vi "I Value (Read).vi"(6 "ISOBUS address":T1=-1 caption="ISOBUS address (-1)", 8 "error in":errorcluster, 11 "Mercury Reference In":T4) -> (0 "error out":errorcluster, 1 "Unit":T2, 2 "I Value":dbl min=0.0 max=100.0 format="%#.1g", 3 "Mercury Reference Out":T4, 4 "Valid?":T3)   [LabVIEW 2013, in "Mercury iXX.lvlib" / "Control Loop.lvlib"]
doc: "Check the I value of the PID associated with control loop."
uses:
  Control Loop.lvlib
  Mercury iXX.lvlib
  Private/Controls/Command Verbs.ctl
  Controls/Unit String.ctl
  Controls/Is Valid LED.ctl
  Controls/Comms Transport Layer.ctl
  Private/Controls/Query Dynamic Reference.ctl
  Controls/Mercury Reference.ctl
  Controls/ISOBus Address.ctl
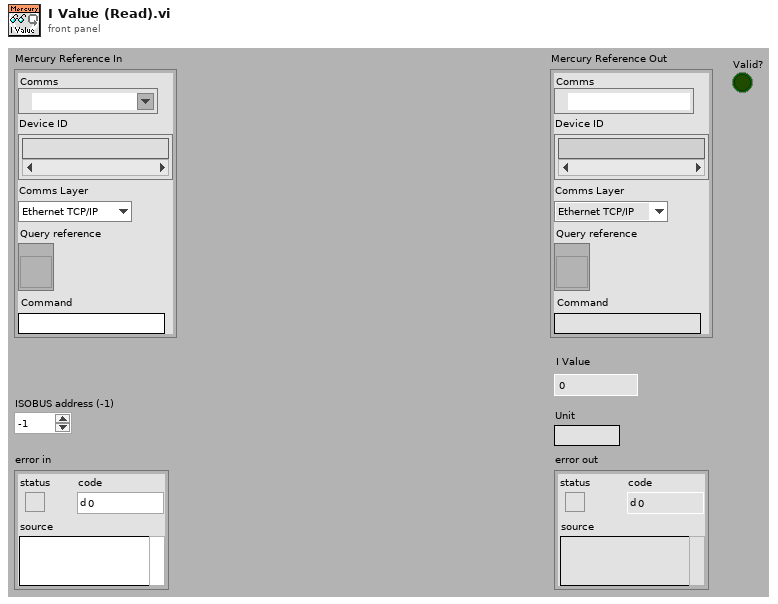
[diagram p1: front panel]
types:
  T1 = typedef "Mercury iXX.lvlib/ISOBus Address.ctl" = i32
  T2 = typedef "Mercury iXX.lvlib/Unit String.ctl" = string
  T3 = typedef "Mercury iXX.lvlib/Is Valid LED.ctl" = bool
  T4 = typedef "Mercury iXX.lvlib/Mercury Reference.ctl" = cluster{"Comms":refnum<visa-resource-name>, "Device ID":string[], "Comms Layer":T5, "Command":string, "Query reference":T6}
  T5 = typedef "Mercury iXX.lvlib/Comms Transport Layer.ctl" = enum16{"Ethernet TCP/IP", "USB", "ISOBus - RS-232", "GPIB"}
  T6 = typedef "Mercury iXX.lvlib/Query Dynamic Reference.ctl" = refnum<vi>
  T7 = typedef "Mercury iXX.lvlib/Command Verbs.ctl" = string
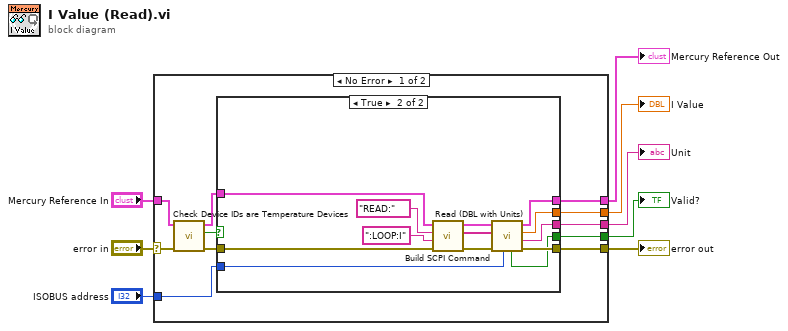
[diagram p0: block diagram]
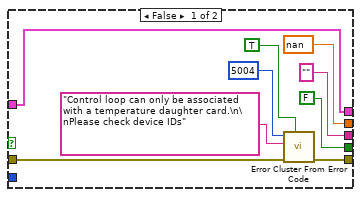
[diagram p2: hidden frame]
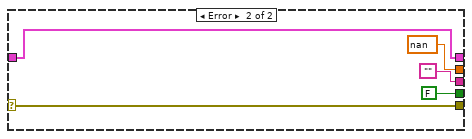
[diagram p3: hidden frame]
diagram:
  n1 = case shown="No Error" "error in" {
    selector: "error in" -> [w15 w45]
    tunnel: "Mercury Reference In" -> [w12 w46]
    tunnel: [w19 w46] -> w1
    tunnel: [w17 w45] -> w5
    tunnel: "ISOBUS address" -> [w18 _]
    tunnel: [w11 nan ("Scaled Value")] -> w2
    tunnel: [w9 FALSE ("Valid?")] -> w4
    tunnel: [w10 ""] -> w3
    frame No Error {
      n2 = call "Check Device IDs are Temperature Devices.vi"("error in"=w15, "Mercury Reference In"=w12) -> ("error out"=w14:errorcluster, "Valid?"=w16:bool, "Mercury Reference Out"=w13:T4)  [unwired: 7 out]
      n3 = case shown="True" w16 {
        tunnel: w13 -> [w28 w37]
        tunnel: [w28 w33] -> w19
        tunnel: w14 -> [w26 w35]
        tunnel: w18 -> [_ w29]
        tunnel: [w27 w34] -> w17
        tunnel: [nan ("Data (Dbl)") w32] -> w11
        tunnel: [T2 "" ("Unit") w31] -> w10
        tunnel: [T3 FALSE ("Valid?") w30] -> w9
        frame False {
          n4 = call <vilib>:"Error Cluster From Error Code.vi"("show call chain? (False)"=TRUE, "error in (no error)"=w26, "error message (\"\")"="Control loop can only be associated with a temperature daughter card.\n\nPlease check device IDs" ("error message (\"\")"), "error code (0)"=5004) -> ("error out"=w27:errorcluster)  [unwired: 5 out]
        }
        frame True {
          n5 = call "Build SCPI Command.vi"("error in"=w35, "Noun(s)"=":LOOP:I" ("Command"), "Verb"=T7 "READ:", "Mercury Reference In"=w37) -> ("error out"=w41:errorcluster, "SCPI Message(s)"=w39:string[], "Mercury Reference Out"=w38:T4)  [unwired: 5 out]
          n6 = call "Read (DBL with Units).vi"("ISOBUS address"=w29, "error in"=w41, "SCPI Message(s)"=w39, "Mercury Reference In"=w38) -> ("error out"=w34:errorcluster, "Unit"=w31:T2, "Data (Dbl)"=w32:dbl, "Mercury Reference Out"=w33:T4, "Valid?"=w30:T3)  [unwired: 3 out]
        }
      }
    }
    frame Error {
    }
  }
  "Mercury Reference Out" <- w1
  "I Value" <- w2
  "Valid?" <- w4
  "Unit" <- w3
  "error out" <- w5
